vi "update_mapid.vi"(10 "input":T1[](array[typedef]) {"Terminal Flags" format="%.0b"}) -> (2 "Output":T1[](array[typedef]) {"Terminal Flags" format="%.0b"})   [LabVIEW 2018]
uses:
  <vilib>/BlockNodeSupport/TerminalData.ctl
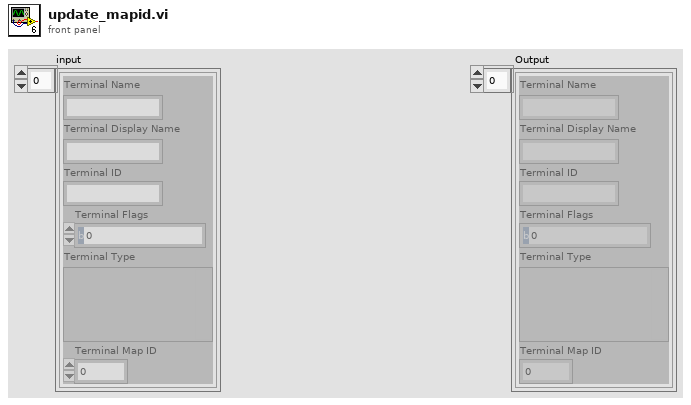
[diagram p1: front panel]
types:
  T1 = typedef "TerminalData.ctl" = cluster{"Terminal Name":string, "Terminal Display Name":string, "Terminal ID":string, "Terminal Flags":i32, "Terminal Type":variant, "Terminal Map ID":i32}
  T2 = enum16{"UPDATE", "READ", "QUERY", "CREATE CHILD", "CREATE", "CONNECT", "DISCONNECT"}
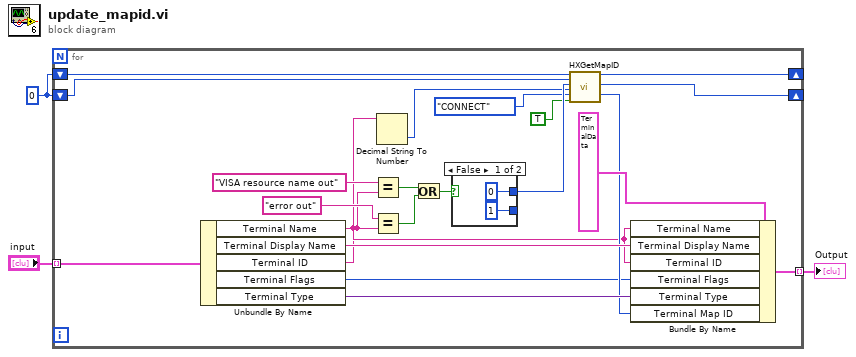
[diagram p0: block diagram]
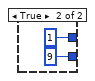
[diagram p2: hidden frame]
diagram:
  w1 = 0 ("input")
  n1 = for {
    tunnel: "input" -> [w23] mode=indexing
    tunnel: [w24] -> w2 mode=indexing
    shift-right: [w20] -> _
    shift-left: w1 -> [w19]
    shift-right: [w18] -> _
    shift-left: w1 -> [w17]
    n2 = Unbundle By Name(w23) -> ("Terminal Name"=w8:string, "Terminal Display Name"=w22:string, "Terminal ID"=w7:string, "Terminal Flags"=w4:i32, "Terminal Type"=w21:variant)
    n3 = Equal?(x="VISA resource name out", y=w8) -> (x = y?=w12:bool)
    n4 = Equal?(x="error out", y=w8) -> (x = y?=w11:bool)
    n5 = Decimal String To Number(string=w7) -> (number=w6:i32)  [unwired: 2 in, 1 out]
    n6 = Or(x=w12, y=w11) -> (x .or. y?=w13:bool)
    n7 = case shown="False" w13 {
      tunnel: [0 ("input") 1 ("input")] -> w10
      tunnel: [1 ("input") 9 ("input")] -> _
      frame False {
      }
      frame True {
      }
    }
    n8 = call <vilib>:"HXGetMapID.vi"("input"=w19, "output"=w17, "direction"=w10, "OldTerm"=w6, "Node type"=T2."CONNECT", "Boolean"=TRUE) -> ("Input"=w20:i32, "Output"=w18:i32, "MapID"=w16:i32)  [unwired: 11 out]
    n9 = Bundle By Name(cluster=T1 {"Terminal Name"="", "Terminal Display Name"="", "Terminal ID"="", "Terminal Flags"=0, "Terminal Type"=variant, "Terminal Map ID"=0} ("input cluster"), "Terminal Name"=w8, "Terminal Display Name"=w22, "Terminal ID"=w8, "Terminal Flags"=w4, "Terminal Type"=w21, "Terminal Map ID"=w16) -> (w24:T1)
  }
  "Output" <- w2
